vi "MICS Command Lookup.vi"(0 "error in":errorcluster, 4 "token":u16) -> (5 "row index":i32=-1, 6 "found":bool, 7 "error out":errorcluster, 8 "tag":string, 9 "command":string)   [LabVIEW 2020]
doc: "This function searches the MICS Command Table indexed by token, to find the corresponding Command and Tag strings.\n\nThe MICS Command Table is inported from SWEX 0085 Rev 1.11, SCS System MICS Commands Design Document, pages 18-21."
panel:
  in  "MICS Commands":string[][](table)=[["1", "0x0001", "Get xPG Status", "TKN_GET_XPG_STATUS"], ["2", "0x0002", "xPG Stimulation", "TKN_XPG_STIMULATION"], ["3", "0x0003", "Select Program", "TKN_SELECT_PROGRAM"], ["4", "0x0004", "Increment Program Amplitude", "TKN_INC_PRGM_AMPL"], ["5", "0x0005", "Decrement Program Amplitude", "TKN_DEC_PRGM_AMPL"], ["6", "0x0006", "Get PoP Constants", "TKN_GET_POP_CONST"], ["7", "0x0007", "Get PPC Constants", "TKN_GET_PPC CONST"], ["8", "0x0008", "Get Program Names", "TKN_GET_PRGM_NAMES"], ["9", "0x0009", "Set Pulse Amplitude", "TKN_SET_PULSE_AMPL"], ["10", "0x000A", "Increment Pulse Amplitude", "TKN_INC_PULSE_AMPL"], ["11", "0x000B", "Decrement Pulse Amplitude", "TKN_DEC_PULSE_AMPL"], ["12", "0x000C", "Get Pulse Widths", "TKN_GET_PULSE_WIDTHS"], ["13", "0x000D", "Set Pulse Widths", "TKN_SET_PULSE_WIDTH"], ["14", "0x000E", "Increment Pulse Width", "TKN_INC_PULSE_WIDTH"], ["15", "0x000F", "Decrement Pulse Width", "TKN_DEC_PULSE_WIDTH"], ["16", "0x0010", "Get Program Frequency", "TKN_GET_PRGM_FREQ"], ["17", "0x0011", "Set Program Frequency", "TKN_SET_PRGM_FREQ"], ["18", "0x0012", "Increment Program Frequency", "TKN_INC_PRGM_FREQ"], ["19", "0x0013", "Decrement Program Frequency", "TKN_DEC_PRGM_FREQ"], ["20", "0x0014", "Inject Event", "TKN_INJECT_EVENT"], ["21", "0x0015", "Charging Control", "TKN_CHARGING_CONTROL"], ["22", "0x0016", "Get xPG Identity", "TKN_GET_XPG_IDENTITY"], ["23", "0x0017", "Set xPG Identity", "TKN_SET_XPG_IDENTITY"], ["24", "0x0018", "Restore Program Defaults", "TKN_RESTORE_DEFAULTS"], ["25", "0x0019", "Get Program Definition", "TKN_GET_PRGM_DEF"], ["26", "0x001A", "Set Program Definition", "TKN_SET_PRGM_DEF"], ["27", "0x001B", "Get Program Constants", "TKN_GET_PRGM_CONST"], ["28", "0x001C", "Set Program Constants", "TKN_SET_PRGM_CONST"], ["29", "0x001D", "Get Configurable Device Parameters", "TKN_GET_CONFIG_PARAMS"], ["30", "0x001E", "Set Configurable Device Parameters", "TKN_SET_CONFIG_PARAMS"], ["31", "0x001F", "Get Pulse Constants", "TKN_GET_PULSE_CONSTANTS"], ["32", "0x0020", "Set Pulse Constants", "TKN_SET_PULSE_CONSTANTS"], ["33", "0x0021", "Get Lead Limits", "TKN_GET_LEAD_LIMITS"], ["34", "0x0022", "Set Lead Limits", "TKN_SET_LEAD_LIMITS"], ["35", "0x0023", "Get Channel Calibrations", "TKN_GET_CHANNEL_CALS"], ["36", "0x0024", "Set Channel Calibrations", "TKN_SET_CHANNEL_CALS"], ["37", "0x0025", "(reserved)", "RESERVED_37"], ["38", "0x0026", "(reserved)", "RESERVED_38"], ["39", "0x0027", "(reserved)", "RESERVED_39"], ["40", "0x0028", "(reserved)", "RESERVED_40"], ["41", "0x0029", "(reserved)", "RESERVED_41"], ["42", "0x002A", "(reserved)", "RESERVED_42"], ["43", "0x002B", "Get Stim Asic HV Calibrations", "TKN_GET_HV_CALS"], ["44", "0x002C", "Set Stim Asic HV Calibrations", "TKN_SET_HV_CALS"], ["45", "0x002D", "(reserved)", "RESERVED_45"], ["46", "0x002E", "(reserved)", "RESERVED_46"], ["47", "0x002F", "Get CP Data", "TKN_GET_CP_DATA"], ["48", "0x0030", "Set CP Data", "TKN_SET_CP_DATA"], ["49", "0x0031", "Clear Log", "TKN_CLEAR_LOG"], ["50", "0x0032", "Read Log", "TKN_READ_LOG"], ["51", "0x0033", "Append Log", "TKN_APPEND_LOG"], ["52", "0x0034", "(reserved)", "RESERVED_52"], ["53", "0x0035", "(reserved)", "RESERVED_53"], ["54", "0x0036", "Impedance Measurement", "TKN_IMP_MEAS"], ["55", "0x0037", "Enter Storage Mode", "TKN_STORAGE"], ["56", "0x0038", "Echo Short", "TKN_ECHO_SHORT"], ["57", "0x0039", "Echo Long", "TKN_ECHO_LONG"], ["58", "0x003A", "Get General Calibration", "TKN_GET_GEN_CAL"], ["59", "0x003B", "Set General Calibration", "TKN_SET_GEN_CAL"], ["60", "0x003C", "Get Trim List", "TKN_GET_TRIM_LIST"], ["61", "0x003D", "Set Trim List", "TKN_SET_TRIM_LIST"], ["62", "0x003E", "Get Counter", "TKN_GET_COUNTER"], ["63", "0x003F", "Set Counter", "TKN_SET_COUNTER"], ["64", "0x0040", "Get Test Stimulation", "TKN_GET_TEST_STIM"], ["65", "0x0041", "Set Test Stimulation", "TKN_SET_TEST_STIM"], ["66", "0x0042", "Get Titration Stimulation", "TKN_GET_TITR_STIM"], ["67", "0x0043", "Set Titration Stimulation", "TKN_SET_TITR_STIM"], ["68", "0x0044", "Get Ramp Time", "TKN_GET_RAMP_TIME"], ["69", "0x0045", "Set Ramp Time", "TKN_SET_RAMP_TIME"], ["70", "0x0046", "Get VBAT", "TKN_GET_VBAT"], ["71", "0x0047", "Set Software Description Block", "TKN_SET_SDB"], ["72", "0x0048", "Get Software Description Block", "TKN_GET_SDB"], ["73", "0x0049", "Write Memory", "TKN_WRITE_MEMORY"], ["74", "0x004A", "Read Memory", "TKN_READ_MEMORY"], ["75", "0x004B", "Reset xPG", "TKN_RESET"], ["76", "0x004C", "Erase Flash Block", "TKN_ERASE_FLASH_BLOCK"], ["77", "0x004D", "Write Vectors", "TKN_WRITE_VECTORS"], ["78", "0x004E", "Read Vectors", "TKN_READ_VECTORS"], ["79", "0x004F", "Diagnostic Data", "TKN_DIAG_DATA"], ["80", "0x0050", "Set Background Impedance", "TKN_SET_BG_IMPEDANCE"], ["81", "0x0051", "Get Background Impedance", "TKN_GET_BG_IMPEDANCE"], ["82", "0x0052", "Set Test Waveform", "TKN_SET_TEST_WAVEFORM"], ["83", "0x0053", "Calibrate Channel", "TKN_CALIBRATE_CHANNEL"], ["84", "0x0054", "Get Log Range", "TKN_GET_LOG_RANGE"], ["85", "0x0055", "(reserved)", "RESERVED_85"], ["86", "0x0056", "(reserved)", "RESERVED_86"], ["87", "0x0057", "MICS Options", "TKN_MICS_OPTIONS"], ["88", "0x0058", "Pair PPC", "TKN_PAIR_PPC"], ["89", "0x0059", "Pair PoP", "TKN_PAIR_POP"], ["90", "0x005A", "Stop Bootloader", "TKN_STOP_BOOTLOADER"], ["91", "0x005B", "Tune MICS", "TKN_MICS_TUNE"], ["92", "0x005C", "MICS Diagnostics", "TKN_MICS_DIAGNOSTICS"], ["32682", "0x7FAA", "Undefined", "TKN_UNDEFINED"]] caption="Table 1"
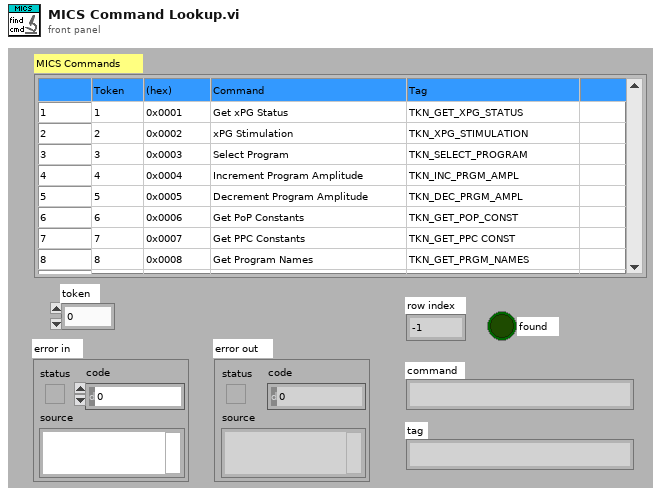
[diagram p1: front panel]
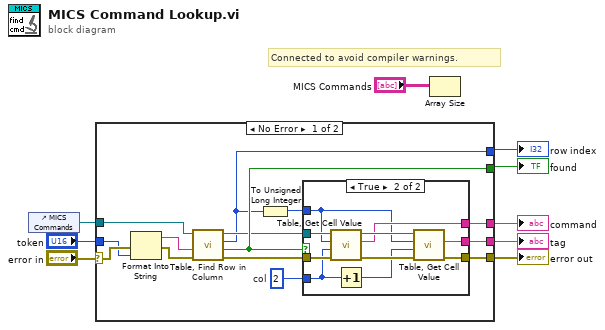
[diagram p0: block diagram]
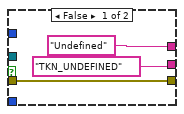
[diagram p2: hidden frame]
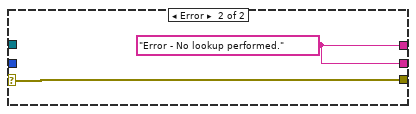
[diagram p3: hidden frame]
diagram:
  # "Connected to avoid compiler warnings."
  n1 = control-ref of="MICS Commands"() -> (w9:refnum<vi>)
  n2 = case shown="No Error" "error in" {
    selector: "error in" -> [w13 w38]
    tunnel: w9 -> [w23 _]
    tunnel: "token" -> [w11 _]
    tunnel: [w21 w38] -> w6
    tunnel: [w20 _] -> w5
    tunnel: [w18 w37] -> w4
    tunnel: [w17 w37] -> w3
    tunnel: [w16 _] -> w2
    frame No Error {
      w14 = u32 2  # col
      n3 = Format Into String(error in=w13, w11) -> (resulting string=w10:string, error out=w12:errorcluster)  [unwired: 2 in]
      n4 = call "Table, Find Row in Column.vi"("error in"=w12, "search key"=w10, "Tbl Refnum"=w23) -> ("error out"=w22:errorcluster, "found"=w20:bool, "row index"=w16:i32, "Tbl Refnum out"=w19:refnum<vi>)  [unwired: 5 in]
      n5 = To Unsigned Long Integer(number=w16) -> (unsigned 32bit integer=w15:u32)
      n6 = case shown="True" w20 {
        tunnel: w22 -> [w26 w36]
        tunnel: [w26 w34] -> w21
        tunnel: w19 -> [_ w33]
        tunnel: ["TKN_UNDEFINED" ("cell value") w31] -> w18
        tunnel: ["Undefined" ("cell value") w30] -> w17
        tunnel: w15 -> [_ w28]
        tunnel: w14 -> [_ w27]
        frame False {
        }
        frame True {
          n7 = call "Table, Get Cell Value.vi"("error in"=w36, "column (0)"=w27, "row (0)"=w28, "Tbl Refnum"=w33) -> ("error out"=w35:errorcluster, "cell value"=w30:string, "Tbl Refnum out"=w32:refnum<vi>)  [unwired: 5 in]
          n8 = Increment(x=w27) -> (x+1=w29:u32)
          n9 = call "Table, Get Cell Value.vi"("error in"=w35, "column (0)"=w29, "row (0)"=w28, "Tbl Refnum"=w32) -> ("error out"=w34:errorcluster, "cell value"=w31:string)  [unwired: 5 in, 1 out]
        }
      }
    }
    frame Error {
      w37 = "Error - No lookup performed." ("cell value")
    }
  }
  "error out" <- w6
  "row index" <- w2
  "found" <- w5
  "command" <- w3
  "tag" <- w4
  n10 = Array Size(array="MICS Commands") -> ()  [unwired: 1 out]
